vi "TagContainerRef To DVR.vi"(1 "TagContainer":T1) -> (0 "DVR":refnum<data-value>)   [LabVIEW 2020, in "TagContainer.lvlib"]
uses:
  TagContainer.lvlib
  Typedef/TagContainer.ctl
  tagcontainer-data.ctl
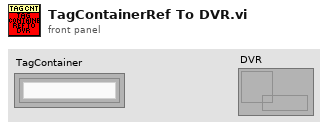
[diagram p1: front panel]
types:
  T1 = typedef "TagContainer.lvlib/TagContainer.ctl" = refnum<k1>
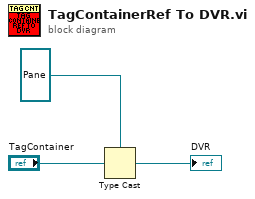
[diagram p0: block diagram]
diagram:
  n1 = Type Cast(type=refnum<data-value> refnum ("data value reference"), x="TagContainer") -> (*(type *) &x=→"DVR":refnum<data-value>)
